vi "main_control_combo_backup.vi"(6 "read":bool=TRUE) -> (9 "chiller readout (temp)":string, 10 "bytes read":u32)   [LabVIEW 2019]
doc: "The Basic Serial Read and Write example performs a Serial Port Read, a Serial Port Write, or a combination of these actions. The user selects the actions (read or write) on the front panel. If both are selected, the VI will write the data first, read data, and then close the VISA session that is opened to the port. This VI will wait until the specified number of bytes is received at the port. Only the number of bytes specified will be read.\n\nINSTRUCTIONS:\n1) Select the serial resource and configuration parameters (baud rate, data bits, parity, stop bits, flow control).\n2) Select the operations to be performed. \n3) Connect the serial port to your device. If no device is available, perform a loopback test by doing one of the following. Short pins 2 and 3 on a RS-232 cable or short pin 4 to pin 8 and pin 5 to pin 9 on a RS-485/422 cable. \n4) Run the VI to see the data read. (The \"read string\" will match the \"string to write\" if a loopback test was performed.)\n\nNote: The parameters set for the serial port must match the parameters of the connected instrument or device. In this example, the bytes to read parameter specifies the number of bytes that the serial port reads. If there were more bytes at the port than the number specified in bytes to read, those bytes would not be read. Also, if you specify to read more bytes than the number of bytes actually read, you might receive a timeout error message.\n\nOn the block diagram, the Configure Serial Port VI sets the configuration parameters. The front panel displays the controls used to configure the basic parameters, such as baud rate, data bits, and parity. Constants configure the other parameters the user probably does not need set. After the VISA Configure Serial Port VI opens the VISA session and configures the port, the VI passes the VISA resource name to other VIs that perform operations on that VISA resource. The VISA Write function sends a command to the serial device and the VISA Read function returns data based on the command. The VISA Close function then closes the reference to the serial device. It is important to close the reference; otherwise communication through with that port through protocols other than VISA might not be possible."
uses:
  <vilib>/Instr/_visa.llb/VISA Configure Serial Port (Instr).vi
  Keithley/Keithley 24XX/Public/Data/Read (Single Point).vi
  <vilib>/Utility/file.llb/Read Delimited Spreadsheet (string).vi
  Keithley/Keithley 24XX/Keithley 24XX.lvlib
  <resource>/objmgr/ni.var.rc
panel:
  in  "read 4":bool
  in  "read \nrotronic log \nmanually":bool
  in  "times to run script":i32
  out "error out":errorcluster
  out "COMBO COMMAND":string
  out "manualDelta":bool
  out "delta readout":string
  in  "delay before read (ms) 4":u32=500
  in  "Combo Box 4":string(combo)
  in  "voltage delta":dbl
  out "delta command":string
  in  "write 4":bool
  in  "stop reading script":bool
  out "dewpoint":string
  out "temperature":string
  out "humidity":string
  out "n2 flow temperature":string
  out "dewpoint":string
  out "From Linux Box":string
  in  "Voltage Manual Range (1.0) 2":dbl=1.0
  in  "Current Manual Range (1.0) 2":dbl=1.0
  in  "Resistance Manual Range (1.0) 2":dbl=1.0
  in  "Enable Voltage Auto Range (T:Enable) 2":bool=TRUE
  in  "Enable Current Auto Range (T:Enable) 2":bool=TRUE
  in  "Enable Resistance Auto Range (T:Enable) 2":bool=TRUE
  out "Voltage 3":sgl
  out "Current 3":sgl
  out "Resistance 2":sgl
  out "Current Micro 2":sgl
  out "Command Log and Output":string
  out "all rows":string[][](array[string])
  out "current command":string[](array[string])
  in  "file path (dialog if empty) 2":path
  in  "Read Script":bool
  out "relay TTi":errorcluster
  out "bytes read 3":u32
  out "inverter readout":string
  in  "read 3":bool=TRUE
  in  "delay before read (ms) 3":u32=500
  in  "Combo Box 3":string(combo)="VO?\n"
  in  "voltage or current 2":dbl
  out "string from combo 3":string
  in  "write 3":bool
  out "LV TTi":errorcluster
  out "bytes read 2":u32
  out "LVPS reaout":string
  in  "read 2":bool=TRUE
  in  "delay before read (ms) 2":u32=500
  in  "Combo Box 2":string(combo)="VO?\n"
  in  "voltage or current":dbl
  in  "write 2":bool
  in  "write":bool
  out "string from combo":string
  in  "Temperature":dbl
  in  "Combo Box":string(combo)
  out "Chiller":errorcluster
  out "N2 temperature > dew point + 5C":bool
  in  "File Path of rotonic datalog":path
  out "time humidity temporature dewpoint":string[](array[string])
  in  "Quit":bool
  in  "delay before read (ms)":u32=500
  # "Kiethley Powersupply"
  # "µA"
  # "Delta powersupply Interface"
  # "TTi LV powersupply Interface for the relay polarity control\nCOM 4 is default"
  # "Medical Chiller Interface\nCOM 6 is default"
  # "TTi LV powersupply Interface\nCOM 5 is default"
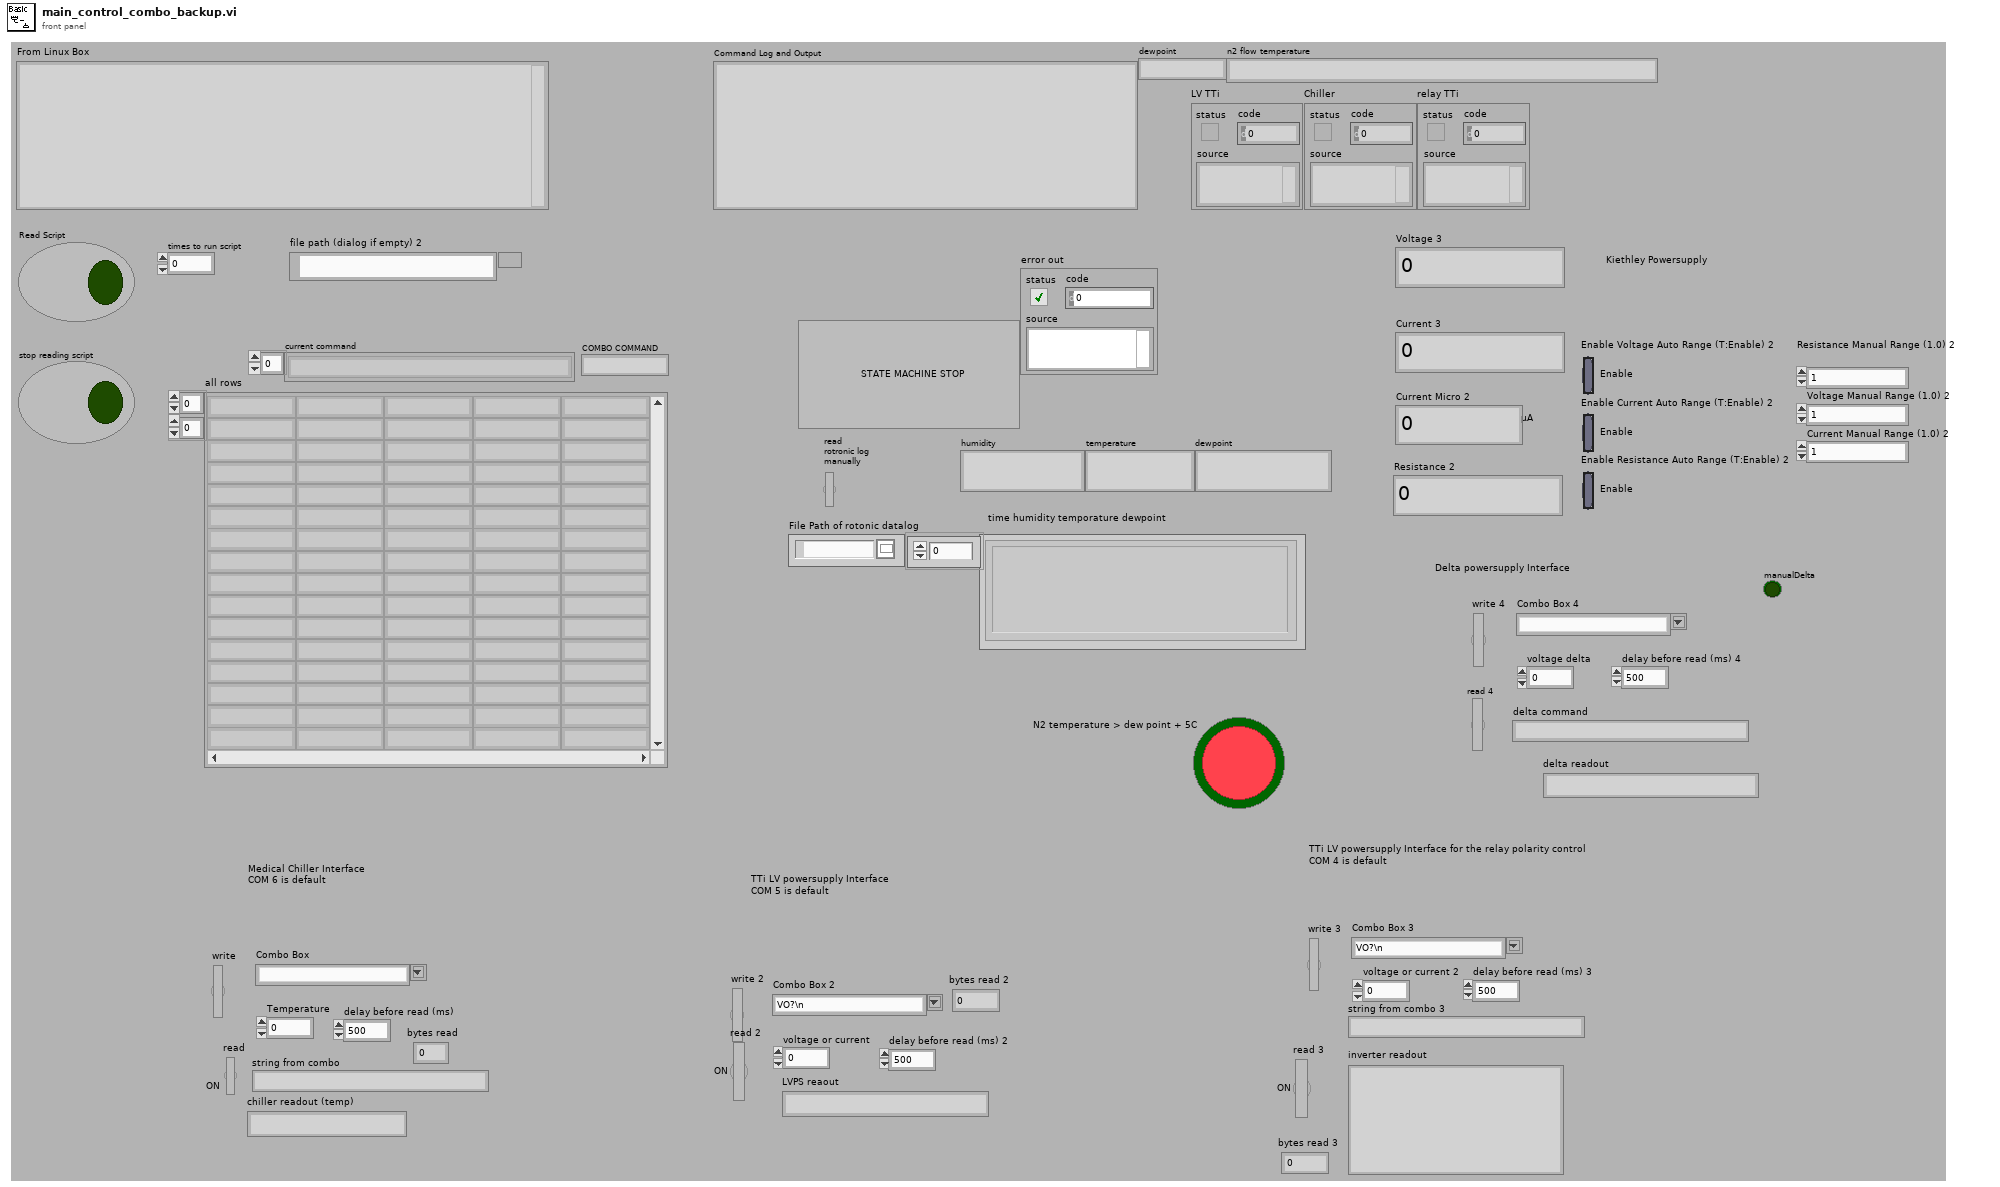
[diagram p1: front panel]
types:
  T1 = cluster{"Baud Rate":u32, "Parity":u16, "Data Bits":u16, "Stop Bits":u16, "Flow Control":u16}
  T2 = enum16{"open", "replace", "create", "open or create", "replace or create", "replace or create with confirmation"}
  T3 = typedef "Semaphore RefNum" = refnum<k1>
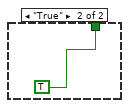
[diagram p2: hidden frame]
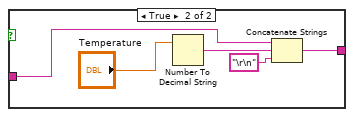
[diagram p5: hidden frame]
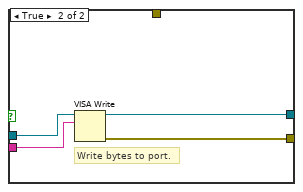
[diagram p6: hidden frame]
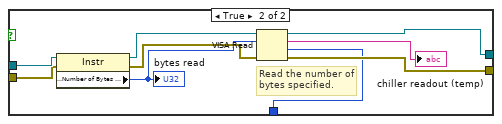
[diagram p7: hidden frame]
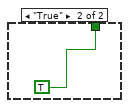
[diagram p8: hidden frame]
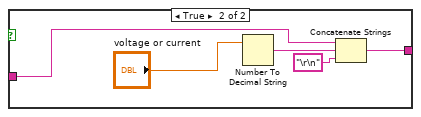
[diagram p10: hidden frame]
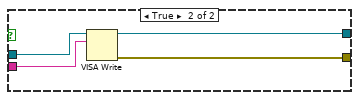
[diagram p11: hidden frame]
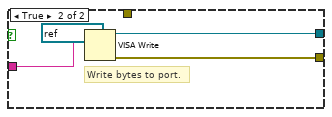
[diagram p16: hidden frame]
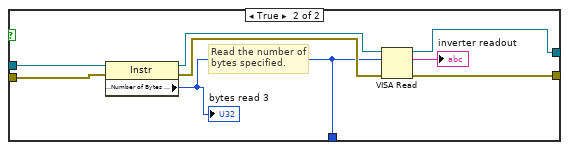
[diagram p17: hidden frame]
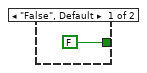
[diagram p18: hidden frame]
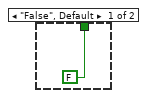
[diagram p19: hidden frame]
diagram:
  # "First save permanent values in non-volatile memory via NI - Max and the *SAV after setting it via SO:VO:MA 52 and SO:CU:MA 30    !"
  n1 = flat-sequence {
    tunnel: [w20] -> w13
    tunnel: [w34] -> w12
    tunnel: [w22] -> w11
    tunnel: [w28] -> w10
    tunnel: [w27] -> w9
    tunnel: [w23] -> w8
    tunnel: [w23] -> w7
    tunnel: [w19] -> w6
    tunnel: [w18] -> w5
    tunnel: [w17] -> w4
    tunnel: [w19] -> w3
    tunnel: [w18] -> w2
    tunnel: [w17] -> w1
    tunnel: [w54] -> w16
    tunnel: [w53] -> w14
    tunnel: w13 -> [w52]
    tunnel: w12 -> [_]
    tunnel: w11 -> [w51]
    tunnel: w10 -> [w49]
    tunnel: w9 -> [w50]
    tunnel: w8 -> [w48]
    tunnel: w7 -> [w47]
    tunnel: w6 -> [w46]
    tunnel: w5 -> [w45]
    tunnel: w4 -> [w44]
    tunnel: w3 -> [w43]
    tunnel: w2 -> [w42]
    tunnel: w1 -> [w41]
    tunnel: w16 -> [w668]
    tunnel: w14 -> [w667]
    frame #0 {
      w21 = refnum<visa-resource-name> "COM4" ("VISA resource name")
      w26 = u32 3000  # timeout (10sec)
      w25 = FALSE  # Enable Termination Char (T)
      w29 = u32 3000  # timeout (10sec)
      w31 = FALSE  # Enable Termination Char (T)
      w32 = u32 3000  # timeout (10sec)
      w35 = FALSE  # Enable Termination Char (T)
      w36 = u32 3000  # timeout (10sec)
      n2 = call "Initialize.vi"("Serial Configuration"=T1 {"Baud Rate"=9600, "Parity"=0, "Data Bits"=8, "Stop Bits"=10, "Flow Control"=1}, "Reset (True)"=FALSE, "VISA resource name"=refnum<visa-resource-name> "COM1" ("VISA resource name 4")) -> ()  [unwired: 7 in, 2 out]
      n3 = local write "COMBO COMMAND"("" ("COMBO COMMAND")) -> ()
      n4 = VISA Open(timeout (0)=w29, VISA resource name=refnum<visa-resource-name> "GPIB0::8::INSTR") -> (VISA resource name=w28:refnum<visa-resource-name>, error out=w27:errorcluster)  [unwired: 3 in]
      n5 = call-poly "VISA Configure Serial Port"("VISA resource name"=refnum<visa-resource-name> "COM5", "timeout (10sec)"=w32, "Enable Termination\nChar (T)"=w31) -> ("VISA resource name out"=w22:refnum<visa-resource-name>)  [unwired: 11 in, 1 out]
      n6 = call <vilib>:"Obtain Semaphore Reference.vi"("name (unnamed)"=w21) -> ("semaphore"=w18:T3)  [unwired: 4 in, 2 out]
      n7 = call-poly "VISA Configure Serial Port"("VISA resource name"=w21, "timeout (10sec)"=w26, "Enable Termination\nChar (T)"=w25) -> ()  [unwired: 11 in, 2 out]
      n8 = call-poly "VISA Configure Serial Port"("VISA resource name"=refnum<visa-resource-name> "COM6", "timeout (10sec)"=w36, "Enable Termination\nChar (T)"=w35) -> ("VISA resource name out"=w20:refnum<visa-resource-name>, "error out"=w34:errorcluster)  [unwired: 11 in]
      n9 = call <vilib>:"Obtain Semaphore Reference.vi"("name (unnamed)"=w22) -> ("semaphore"=w17:T3)  [unwired: 4 in, 2 out]
      n10 = call <vilib>:"Obtain Semaphore Reference.vi"("name (unnamed)"=w20) -> ("semaphore"=w19:T3)  [unwired: 4 in, 2 out]
      n11 = call <vilib>:"Obtain Semaphore Reference.vi"("name (unnamed)"=w28) -> ("semaphore"=w23:T3)  [unwired: 4 in, 2 out]
    }
    frame #1 {
      # "Disable Output"
      # "State machine for iterating through commands from table"
      n12 = while {
        tunnel: w48 -> [w367]
        tunnel: w46 -> [w366]
        tunnel: w45 -> [w365]
        tunnel: w44 -> [w364]
        stop <- w369 stop-if-true
        # "LV TTi SEH"
        # "inverter"
        # "chiller"
        # "DeltaRef"
        n13 = local read "Quit"() -> (w369:bool)
        n14 = case shown="True" "Read Script" {
          tunnel: "times to run script" -> [_ w375]
          tunnel: w367 -> [_ w374]
          tunnel: w366 -> [_ w373]
          tunnel: w365 -> [_ w372]
          tunnel: w364 -> [_ w371]
          frame False {
          }
          frame True {
            n15 = Get Date/Time String() -> (date string=w398:string, time string=w396:string)  [unwired: 3 in]
            n16 = Search and Replace String(replace all?=TRUE ("replace all? (F)"), input string=w398, search string="/", replace string="_" ("replace string (\"\")")) -> (result string=w397:string)  [unwired: 4 in, 3 out]
            n17 = Search and Replace String(input string=w396, search string=":", replace string="" ("replace string (\"\")")) -> (result string=w395:string)  [unwired: 5 in, 3 out]
            n18 = Concatenate Strings("C:\\Users\\CMSOTDSF.CERN\\ExecutedCommands\\" ("string"), "command_log_" ("string"), w397, "_" ("string"), w395, ".txt" ("string")) -> (w394:string)
            n19 = String To Path(string=w394) -> (path=w384:path)
            n20 = Open/Create/Replace File(file path (use dialog)=w384, operation (0:open)=T2."replace or create") -> (refnum out=w383:refnum<file>)  [unwired: 4 in, 2 out]
            n21 = Concatenate Strings("Command Log Header for Executed CSV commands " ("text"), "\r\n") -> (w376:string)
            n22 = Set File Position(offset (in bytes) (0)=i64 0, refnum=w383, from (0:start)=enum16{"start", "end", "current"}."end") -> (refnum out=w380:refnum<file>)  [unwired: 1 in, 1 out]
            n23 = Write to Text File(file (use dialog)=w380, text=w376) -> ()  [unwired: 2 in, 3 out]
            n24 = flat-sequence {
              tunnel: w384 -> [w404]
              tunnel: w375 -> [w403]
              tunnel: w374 -> [w402]
              tunnel: w373 -> [w401]
              tunnel: w372 -> [w400]
              tunnel: w371 -> [w399]
              frame #0 {
                n25 = for {
                  N: w403 -> [_]
                  tunnel: w404 -> [w409]
                  tunnel: w402 -> [w408]
                  tunnel: w401 -> [w407]
                  tunnel: w400 -> [w406]
                  tunnel: w399 -> [w405]
                  n26 = flat-sequence {
                    tunnel: ["file path (dialog if empty) 2"] -> w412
                    tunnel: [w415] -> w411
                    tunnel: [w413] -> w410
                    tunnel: w409 -> [w413]
                    tunnel: w412 -> [_]
                    tunnel: w411 -> [w422]
                    tunnel: w410 -> [w421]
                    tunnel: w408 -> [w420]
                    tunnel: w407 -> [w419]
                    tunnel: w406 -> [w418]
                    tunnel: w405 -> [w417]
                    frame #0 {
                      # "read table from CSV"
                      n27 = call-poly <vilib>:"Read Delimited Spreadsheet.vi"("file path (dialog if empty)"="file path (dialog if empty) 2", "delimiter (\\t)"="," ("delimiter (\\t)")) -> ("all rows"=w415:string[][])  [unwired: 8 in, 5 out]
                    }
                    frame #1 {
                      n28 = Array Size(array=w422) -> (size(s)=w425:i32[])
                      n29 = Index Array(array=w425, index #1=0 ("index"), index #2=1 ("index")) -> (element #1=w426:i32)  [unwired: 1 out]
                      n30 = for {
                        N: w426 -> [_]
                        tunnel: w422 -> [w454] mode=indexing
                        tunnel: w421 -> [w442]
                        tunnel: w420 -> [w430]
                        tunnel: w419 -> [w429]
                        tunnel: w418 -> [w428]
                        tunnel: w417 -> [w427]
                        i -> [w439]
                        stop <- w448 stop-if-true
                        n31 = local read "Quit"() -> (w450:bool)
                        n32 = Array Subset(array=w454) -> (w451:string[])  [unwired: 2 in]
                        "current command" <- w451
                        n33 = Or(x=w450, y="stop reading script") -> (x .or. y?=w448:bool)
                        n34 = Array Size(array=w451) -> (size(s)=w453:i32)
                        n35 = Index Array(array=w451, index=0) -> (element=w431:string)
                        "COMBO COMMAND" <- w431
                        n36 = for {
                          N: w453 -> [_]
                          tunnel: w451 -> [w614]
                          tunnel: [w615] -> w432 mode=indexing
                          i -> [w617]
                          n37 = Add(x=w617, y=1) -> (x+y=w613:i32)
                          n38 = Index Array(array=w614, index=w613) -> (element=w612:string)
                          n39 = Wait Until Next ms Multiple(millisecond multiple=u32 1000) -> ()  [unwired: 1 out]
                          n40 = Concatenate Strings(w612, "   " ("string")) -> (w615:string)
                        }
                        n41 = case shown="\"setDeltaPS\"" w431 {
                          tunnel: w451 -> [w462 w474 w495 w513 w548 w576 _ _]
                          tunnel: [w455 w471 w493 w505 w541 w572 _ w585] -> w440
                          tunnel: w430 -> [_ _ w487 w504 _ _ _ _]
                          tunnel: w429 -> [_ _ _ _ w540 _ _ _]
                          tunnel: w428 -> [_ _ _ w500 _ _ _ _]
                          tunnel: w427 -> [_ w463 _ _ _ _ _ _]
                          frame "wait", Default {
                            n42 = Array Subset(array=w462, index=1) -> (w460:string[])  [unwired: 1 in]
                            n43 = Index Array(array=w460, index=0) -> (element=w456:string)
                            n44 = Decimal String To Number(string=w456) -> (number=w458:i32)  [unwired: 2 in, 1 out]
                            n45 = Wait (ms)(milliseconds to wait=w458) -> ()  [unwired: 1 out]
                            n46 = Concatenate Strings("Wait for ", w456) -> (w455:string)
                          }
                          frame "setLVPS" {
                            # "Write bytes to port."
                            # "MUST specify codes display with single \"\\\""
                            # "Configure Serial port (baud rate,\ndata bits, parity, stop bits and flow control)."
                            n47 = Array Subset(array=w474, index=1) -> (w479:string[])  [unwired: 1 in]
                            n48 = Index Array(array=w479, index #1=0 ("index"), index #2=1 ("index")) -> (element #1=w476:string)  [unwired: 1 out]
                            n49 = Decimal String To Number(string=w476) -> (number=w473:i32)  [unwired: 2 in, 1 out]
                            n50 = To Double Precision Float(number=w473) -> (double precision float=w470:dbl)
                            n51 = case shown="0, Default" w470 {
                              tunnel: ["OP 0\n" ("Combo Box 4") "OP 1\n" ("Combo Box 4")] -> w469
                              tunnel: ["0" ("Combo Box 4") "11" ("Combo Box 4")] -> w467
                              frame 0, Default {
                              }
                              frame 1 {
                              }
                            }
                            n52 = call <vilib>:"Acquire Semaphore.vi"("semaphore"=w463) -> ("error out"=w465:errorcluster, "semaphore out"=w466:T3)  [unwired: 4 in, 1 out]
                            n53 = VISA Write(VISA resource name=refnum<visa-resource-name> "COM5", write buffer=w469, error in (no error)=w465) -> (error out=w464:errorcluster)  [unwired: 2 out]
                            n54 = call <vilib>:"Release Semaphore.vi"("error in (no error)"=w464, "semaphore"=w466) -> ()  [unwired: 4 in, 2 out]
                            n55 = Concatenate Strings("we just set the LV PS voltage to ", w467) -> (w471:string)
                          }
                          frame "setDeltaPS" {
                            # "MUST specify codes display with single \"\\\""
                            # "Configure Serial port (baud rate,\ndata bits, parity, stop bits and flow control)."
                            n56 = Array Subset(array=w495, index=1) -> (w499:string[])  [unwired: 1 in]
                            n57 = Index Array(array=w499, index #1=0 ("index"), index #2=1 ("index")) -> (element #1=w488:string)  [unwired: 1 out]
                            n58 = call <vilib>:"Acquire Semaphore.vi"("semaphore"=w487) -> ("error out"=w486:errorcluster, "semaphore out"=w484:T3)  [unwired: 4 in, 1 out]
                            n59 = Concatenate Strings("SOUR:VO " ("format string"), w488, "\n" ("string")) -> (w490:string)
                            n60 = VISA Write(VISA resource name=refnum<visa-resource-name> "GPIB0::8::INSTR", write buffer=w490, error in (no error)=w486) -> (error out=w485:errorcluster)  [unwired: 2 out]
                            n61 = call <vilib>:"Release Semaphore.vi"("error in (no error)"=w485, "semaphore"=w484) -> ()  [unwired: 4 in, 2 out]
                            n62 = Concatenate Strings("we just set the Delta voltage to ", w488) -> (w493:string)
                          }
                          frame "setInverter" {
                            # "MUST specify codes display with single \"\\\""
                            # "Configure Serial port (baud rate,\ndata bits, parity, stop bits and flow control)."
                            n63 = Array Subset(array=w513, index=1) -> (w518:string[])  [unwired: 1 in]
                            n64 = Index Array(array=w518, index #1=0 ("index"), index #2=1 ("index")) -> (element #1=w515:string)  [unwired: 1 out]
                            n65 = Decimal String To Number(string=w515) -> (number=w512:i32)  [unwired: 2 in, 1 out]
                            n66 = To Double Precision Float(number=w512) -> (double precision float=w506:dbl)
                            n67 = call <vilib>:"Acquire Semaphore.vi"("semaphore"=w504) -> ("error out"=w503:errorcluster, "semaphore out"=w501:T3)  [unwired: 4 in, 1 out]
                            n68 = call "deltaPS.vi"("error in (no error)"=w503, "VISA Refnum in"=refnum<visa-resource-name> "GPIB0::8::INSTR" ("VISA resource name")) -> ("error out"=w502:errorcluster, "DeltaPS"=w507:string)  [unwired: 8 in]
                            n69 = Decimal String To Number(string=w507) -> (number=w508:i32)  [unwired: 2 in, 1 out]
                            n70 = Less?(x=w508, y=3.0) -> (x < y?=w510:bool)
                            n71 = case shown="False" w510 {
                              tunnel: w506 -> [_ w530]
                              tunnel: w507 -> [w521 _]
                              tunnel: [w520 w527] -> w505
                              tunnel: w500 -> [_ w523]
                              frame False {
                                n72 = local write "stop reading script"(TRUE ("stop reading script")) -> ()
                                n73 = Concatenate Strings("Dangerous polarity switching   Delta PS too high:    ", w521) -> (w520:string)
                                n74 = call "Send Email"("Message"=w520) -> ()  [unwired: 10 in, 1 out]
                              }
                              frame True {
                                # "Write bytes to port."
                                n75 = case shown="1" w530 {
                                tunnel: ["OP 0\n" ("Combo Box 4") "OP 1\n" ("Combo Box 4")] -> w532
                                tunnel: ["0" ("Combo Box 4") "10" ("Combo Box 4")] -> w528
                                frame 0, Default {
                                }
                                frame 1 {
                                }
                                }
                                n76 = call <vilib>:"Acquire Semaphore.vi"("semaphore"=w523) -> ("error out"=w526:errorcluster, "semaphore out"=w524:T3)  [unwired: 4 in, 1 out]
                                n77 = VISA Write(VISA resource name=refnum<visa-resource-name> "COM4", write buffer=w532, error in (no error)=w526) -> (error out=w525:errorcluster)  [unwired: 2 out]
                                n78 = Concatenate Strings("we just set the Inverter voltage to ", w528) -> (w527:string)
                                n79 = call <vilib>:"Release Semaphore.vi"("error in (no error)"=w525, "semaphore"=w524) -> ()  [unwired: 4 in, 2 out]
                              }
                            }
                            n80 = call <vilib>:"Release Semaphore.vi"("error in (no error)"=w502, "semaphore"=w501) -> ()  [unwired: 4 in, 2 out]
                          }
                          frame "setChiller" {
                            # "Write bytes to port."
                            # "MUST specify codes display with single \"\\\""
                            # "Configure Serial port (baud rate,\ndata bits, parity, stop bits and flow control)."
                            n81 = Array Subset(array=w548, index=1) -> (w552:string[])  [unwired: 1 in]
                            n82 = Index Array(array=w552, index #1=0 ("index"), index #2=1 ("index")) -> (element #1=w543:string, element #2=w545:string)
                            n83 = Decimal String To Number(string=w545) -> (number=w544:i32)  [unwired: 2 in, 1 out]
                            n84 = To Double Precision Float(number=w544) -> (double precision float=w542:dbl)
                            n85 = call <vilib>:"Acquire Semaphore.vi"("semaphore"=w540) -> ("error out"=w539:errorcluster, "semaphore out"=w538:T3)  [unwired: 4 in, 1 out]
                            n86 = case shown="\"stop\", Default" w543 {
                              tunnel: ["STOP\n" ("Combo Box 4") "START\n" ("Combo Box 4") w561] -> w547
                              tunnel: w542 -> [_ _ w560]
                              tunnel: ["we just stop the chiller" "we just start the chiller" w557] -> w541
                              frame "stop", Default {
                              }
                              frame "start" {
                              }
                              frame "settemp" {
                                n87 = Number To Decimal String(number=w560) -> (decimal integer string=w559:string)  [unwired: 1 in]
                                n88 = Concatenate Strings("OUT_SP_00_" ("Combo Box 4"), w559, "\r\n" ("string")) -> (w561:string)
                                n89 = Concatenate Strings("we just set the Chiller temperature to ", w559) -> (w557:string)
                              }
                            }
                            n90 = VISA Write(VISA resource name=refnum<visa-resource-name> "COM6", write buffer=w547, error in (no error)=w539) -> (error out=w537:errorcluster)  [unwired: 2 out]
                            n91 = call <vilib>:"Release Semaphore.vi"("error in (no error)"=w537, "semaphore"=w538) -> ()  [unwired: 4 in, 2 out]
                          }
                          frame "keithleynew" {
                            w564 = u16 0 items=["Voltage", "Current"] ("Source Mode  (0: Voltage)")
                            # "Configure each of the three measurements. settings"
                            n92 = Array Subset(array=w576, index=1) -> (w579:string[])  [unwired: 1 in]
                            n93 = Index Array(array=w579, index #1=0 ("index"), index #2=1 ("index")) -> (element #1=w573:string)  [unwired: 1 out]
                            n94 = Decimal String To Number(string=w573) -> (number=w575:i32)  [unwired: 2 in, 1 out]
                            n95 = To Double Precision Float(number=w575) -> (double precision float=w570:dbl)
                            n96 = Concatenate Strings("we just set the keithley voltage to ", w573) -> (w572:string)
                            n97 = call "Configure Output.vi"("Source Mode  (0: Voltage)"=w564, "Compliance  Level (0.1)"=1e-05, "Output Level (0)"=w570, "VISA resource name"=refnum<visa-resource-name> "COM1") -> ("error out"=w568:errorcluster, "VISA resource name out"=w569:refnum<visa-resource-name>)  [unwired: 6 in]
                            n98 = call "Enable Output.vi"("error in (no error)"=w568, "Enable Output (T: Enable)"=TRUE, "VISA resource name"=w569) -> ()  [unwired: 7 in, 2 out]
                          }
                          frame "closekeithley" {
                            n99 = call "Enable Output.vi"("Enable Output (T: Enable)"=FALSE, "VISA resource name"=refnum<visa-resource-name> "COM1") -> ("error out"=w581:errorcluster, "VISA resource name out"=w582:refnum<visa-resource-name>)  [unwired: 8 in]
                            n100 = call "Close.vi"("error in (no error)"=w581, "VISA resource name"=w582) -> ("error out"=w584:errorcluster)  [unwired: 9 in]
                            n101 = call <vilib>:"Simple Error Handler.vi"("error in (no error)"=w584) -> ()  [unwired: 4 in, 5 out]
                          }
                          frame "2sCalibration" {
                            # "C:\\Users\\CMSOTDSF.CERN\\2sCalibrationOut"
                            # "run a windows batch file that will call ssh command with an INPUT bash script\nThe input bash script will run the 2s calibration and is located here:\nC:\\Users\\CMSOTDSF.CERN\\cc7.sh"
                            n102 = flat-sequence {
                              tunnel: [w588] -> w586
                              tunnel: w586 -> [w594]
                              tunnel: [w593] -> w585
                              frame #0 {
                                n103 = call <vilib>:"System Exec.vi"("run minimized? (F)"=TRUE, "working directory"=path "C:/Users/CMSOTDSF.CERN/OpenSSH", "command line"="cmd /c C:\\Users\\CMSOTDSF.CERN\\windows_cc7.bat") -> ("standard error"=w589:string, "standard output"=w590:string)  [unwired: 5 in, 2 out]
                                "From Linux Box" <- w590
                                n104 = Concatenate Strings(w590, w589) -> (w588:string)
                              }
                              frame #1 {
                                n105 = Get Date/Time String() -> (date string=w605:string, time string=w607:string)  [unwired: 3 in]
                                n106 = Search and Replace String(input string=w607, search string=":", replace string="" ("replace string (\"\")")) -> (result string=w608:string)  [unwired: 5 in, 3 out]
                                n107 = Search and Replace String(replace all?=TRUE ("replace all? (F)"), input string=w605, search string="/", replace string="_" ("replace string (\"\")")) -> (result string=w606:string)  [unwired: 4 in, 3 out]
                                n108 = Concatenate Strings("C:\\Users\\CMSOTDSF.CERN\\2sCalibrationOut\\" ("string"), "2scalibration_" ("string"), w606, "_" ("string"), w608, ".txt" ("string")) -> (w609:string)
                                n109 = String To Path(string=w609) -> (path=w610:path)
                                n110 = Concatenate Strings("2S Calibration done output is saved to: ", w609) -> (w593:string)
                                n111 = Write to Text File(file (use dialog)=w610, text=w594) -> ()  [unwired: 2 in, 3 out]
                              }
                            }
                          }
                        }
                        "Command Log and Output" <- w440
                        n112 = Add(x=w439, y=1) -> (x+y=w437:i32)
                        n113 = Number To Decimal String(number=w437) -> (decimal integer string=w436:string)  [unwired: 1 in]
                        n114 = Open/Create/Replace File(file path (use dialog)=w442, operation (0:open)=T2."open") -> (refnum out=w443:refnum<file>)  [unwired: 4 in, 2 out]
                        n115 = Concatenate Strings(w436, "  " ("string"), w431, "  " ("string"), w432, "\r\n") -> (w441:string)
                        n116 = Set File Position(offset (in bytes) (0)=i64 0, refnum=w443, from (0:start)=enum16{"start", "end", "current"}."end") -> (refnum out=w445:refnum<file>)  [unwired: 1 in, 1 out]
                        n117 = Write to Text File(file (use dialog)=w445, text=w441) -> ()  [unwired: 2 in, 3 out]
                      }
                      "all rows" <- w422
                    }
                  }
                }
              }
              frame #1 {
                n118 = local write "COMBO COMMAND"("" ("COMBO COMMAND")) -> ()
                n119 = invoke on="Read Script" class="Bool (strict)" method="Reinit To Default"() -> ()  [unwired: 3 in, 3 out]
                n120 = invoke on="stop reading script" class="Bool (strict)" method="Reinit To Default"() -> ()  [unwired: 3 in, 3 out]
              }
            }
          }
        }
      }
      n121 = while {
        tunnel: w49 -> [_]
        tunnel: w50 -> [_]
        tunnel: w47 -> [w253]
        stop <- w267 stop-if-true
        w256 = "True" ("replace string (\"\")")
        n122 = local read "COMBO COMMAND"() -> (w260:string)
        n123 = Search and Replace String(input string=w260, search string="setInverter", replace string=w256) -> (result string=w265:string)  [unwired: 5 in, 3 out]
        n124 = Search and Replace String(input string=w260, search string="setDeltaPS", replace string=w256) -> (result string=w262:string)  [unwired: 5 in, 3 out]
        n125 = case shown="\"True\"" w265 {
          tunnel: [FALSE TRUE] -> w266
          frame "False", Default {
          }
          frame "True" {
          }
        }
        n126 = case shown="\"False\", Default" w262 {
          tunnel: [FALSE TRUE] -> w263
          frame "False", Default {
          }
          frame "True" {
          }
        }
        n127 = local read "Quit"() -> (w264:bool)
        n128 = call <vilib>:"Acquire Semaphore.vi"("semaphore"=w253) -> ("error out"=w254:errorcluster, "semaphore out"=w251:T3)  [unwired: 4 in, 1 out]
        n129 = Or(x=w263, y=w264) -> (x .or. y?=w259:bool)
        n130 = Or(x=w259, y=w266) -> (x .or. y?=w258:bool)
        n131 = Not(x=w258) -> (.not. x?=w261:bool)
        "manualDelta" <- w261
        n132 = case shown="True" w261 {
          tunnel: w254 -> [w270 w276]
          tunnel: [w270 w275] -> w252
          frame False {
          }
          frame True {
            # "delta"
            # "Configure Serial port (baud rate,\ndata bits, parity, stop bits and flow control)."
            n133 = Match True/False String(2:"" ("false string"), 3:"SOUR:VO " ("format string"), 4:"Combo Box 4") -> (0:w281:bool)  [unwired: 1 out]
            n134 = case shown="True" w281 {
              tunnel: [w289 w292] -> w278
              tunnel: "Combo Box 4" -> [w289 w291]
              frame False {
              }
              frame True {
                n135 = Number To Decimal String(number="voltage delta") -> (decimal integer string=w294:string)  [unwired: 1 in]
                n136 = Concatenate Strings(w291, w294, "\n" ("string")) -> (w292:string)
              }
            }
            "delta command" <- w278
            n137 = case shown="True" "write 4" {
              tunnel: [w300 w306] -> w286
              tunnel: [w301 w305] -> w284
              tunnel: w278 -> [_ w304]
              tunnel: w276 -> [w298 _]
              frame False {
                n138 = VISA Write(VISA resource name=refnum<visa-resource-name> "GPIB0::8::INSTR", write buffer="ME:VO?\n", error in (no error)=w298) -> (VISA resource name out=w301:refnum<visa-resource-name>, error out=w300:errorcluster)  [unwired: 1 out]
              }
              frame True {
                # "Write bytes to port."
                n139 = VISA Write(VISA resource name=refnum<visa-resource-name> "GPIB0::8::INSTR", write buffer=w304) -> (VISA resource name out=w305:refnum<visa-resource-name>, error out=w306:errorcluster)  [unwired: 1 in, 1 out]
              }
            }
            n140 = stacked-sequence {
              tunnel: w286 -> [w297]
              tunnel: [w297] -> w285
              tunnel: w284 -> [w296]
              tunnel: [w296] -> w283
              frame #0 {
                n141 = Wait (ms)(milliseconds to wait="delay before read (ms) 4") -> ()  [unwired: 1 out]
              }
            }
            n142 = case shown="True" "read 4" {
              tunnel: w285 -> [w309 w311]
              tunnel: [w309 w316] -> w275
              tunnel: [w308 w315] -> _
              tunnel: w283 -> [w308 w313]
              tunnel: [u32 10 ("return count") w310] -> w273
              frame False {
              }
              frame True {
                # "Read the number of bytes specified."
                n143 = VISA Read(VISA resource name=w313, byte count=u32 1024, error in (no error)=w311) -> (VISA resource name out=w315:refnum<visa-resource-name>, read buffer=→"delta readout":string, return count=w310:u32, error out=w316:errorcluster)
              }
            }
            n144 = Equal?(x=w273, y=0.0) -> (x = y?=w272:bool)
            n145 = case shown="True" w272 {
              frame False {
              }
              frame True {
                n146 = call "delta email"() -> ()  [unwired: 11 in, 1 out]
                n147 = local write "stop reading script"(TRUE ("stop reading script")) -> ()
                n148 = local write "write 4"(TRUE ("write 4")) -> ()
              }
            }
          }
        }
        n149 = local read "Quit"() -> (w267:bool)
        n150 = call <vilib>:"Release Semaphore.vi"("error in (no error)"=w252, "semaphore"=w251) -> ()  [unwired: 4 in, 2 out]
      }
      n151 = while {
        stop <- "Quit" stop-if-true
      }
      n152 = while {
        tunnel: w51 -> [w139]
        tunnel: [w140] -> w54
        tunnel: w41 -> [w128]
        stop <- w138 stop-if-true
        n153 = local read "COMBO COMMAND"() -> (w130:string)
        n154 = call <vilib>:"Acquire Semaphore.vi"("semaphore"=w128) -> ("error out"=w127:errorcluster, "semaphore out"=w125:T3)  [unwired: 4 in, 1 out]
        n155 = Search and Replace String(input string=w130, search string="setLVPS", replace string="True" ("replace string (\"\")")) -> (result string=w135:string)  [unwired: 5 in, 3 out]
        n156 = case shown="\"False\", Default" w135 {
          tunnel: [FALSE TRUE] -> w136
          frame "False", Default {
          }
          frame "True" {
          }
        }
        n157 = local read "Quit"() -> (w137:bool)
        n158 = Or(x=w136, y=w137) -> (x .or. y?=w132:bool)
        n159 = Not(x=w132) -> (.not. x?=w131:bool)
        n160 = case shown="True" w131 {
          tunnel: [w143 w159] -> w126
          tunnel: [w144 w158] -> w140
          tunnel: w139 -> [w144 w157]
          tunnel: w127 -> [w143 w145]
          frame False {
          }
          frame True {
            # "TTi SEH PS LV"
            n161 = Match True/False String(2:"" ("false string"), 3:"OUT_SP_00_" ("format string"), 4:"Combo Box 2") -> (0:w150:bool)  [unwired: 1 out]
            n162 = case shown="False" w150 {
              tunnel: [w160 w163] -> w147
              tunnel: "Combo Box 2" -> [w160 w162]
              frame False {
              }
              frame True {
                n163 = Number To Decimal String(number="voltage or current") -> (decimal integer string=w165:string)  [unwired: 1 in]
                n164 = Concatenate Strings(w162, w165, "\r\n" ("string")) -> (w163:string)
              }
            }
            n165 = case shown="False" "write 2" {
              tunnel: [w170 w177] -> w155
              tunnel: w157 -> [w172 w176]
              tunnel: [w171 w175] -> w153
              tunnel: w147 -> [_ w174]
              tunnel: w145 -> [w169 _]
              frame False {
                n166 = VISA Write(VISA resource name=w172, write buffer="VO?\n", error in (no error)=w169) -> (VISA resource name out=w171:refnum<visa-resource-name>, error out=w170:errorcluster)  [unwired: 1 out]
              }
              frame True {
                n167 = VISA Write(VISA resource name=w176, write buffer=w174) -> (VISA resource name out=w175:refnum<visa-resource-name>, error out=w177:errorcluster)  [unwired: 1 in, 1 out]
              }
            }
            n168 = stacked-sequence {
              tunnel: w155 -> [w168]
              tunnel: [w168] -> w154
              tunnel: w153 -> [w167]
              tunnel: [w167] -> w152
              frame #0 {
                n169 = Wait (ms)(milliseconds to wait="delay before read (ms) 2") -> ()  [unwired: 1 out]
              }
            }
            n170 = case shown="True" "read 2" {
              tunnel: w154 -> [w179 w183]
              tunnel: [w179 w187] -> w159
              tunnel: [w178 w186] -> w158
              tunnel: w152 -> [w178 w185]
              frame False {
              }
              frame True {
                # "Read the number of bytes specified."
                n171 = property class="Instr"(reference=w185, error in=w183) -> (reference out=w184:refnum<visa-resource-name>, error out=w182:errorcluster, "Serial Settings:Number of Bytes at Serial Port"=w181:u32)
                "bytes read 2" <- w181
                n172 = VISA Read(VISA resource name=w184, byte count=w181, error in (no error)=w182) -> (VISA resource name out=w186:refnum<visa-resource-name>, read buffer=→"LVPS reaout":string, error out=w187:errorcluster)  [unwired: 1 out]
              }
            }
          }
        }
        n173 = call <vilib>:"Release Semaphore.vi"("error in (no error)"=w126, "semaphore"=w125) -> ()  [unwired: 4 in, 2 out]
        n174 = local read "Quit"() -> (w138:bool)
        n175 = Wait Until Next ms Multiple(millisecond multiple=u32 1000) -> ()  [unwired: 1 out]
      }
      n176 = while {
        tunnel: w42 -> [w191]
        stop <- w200 stop-if-true
        # "TTi Inverter for Relay"
        n177 = local read "COMBO COMMAND"() -> (w198:string)
        n178 = call <vilib>:"Acquire Semaphore.vi"("semaphore"=w191) -> ("error out"=w188:errorcluster, "semaphore out"=w190:T3)  [unwired: 4 in, 1 out]
        n179 = Search and Replace String(input string=w198, search string="setInverter", replace string="True" ("replace string (\"\")")) -> (result string=w194:string)  [unwired: 5 in, 3 out]
        n180 = case shown="\"True\"" w194 {
          tunnel: [FALSE TRUE] -> w195
          frame "False", Default {
          }
          frame "True" {
          }
        }
        n181 = local read "Quit"() -> (w196:bool)
        n182 = Or(x=w195, y=w196) -> (x .or. y?=w197:bool)
        n183 = Not(x=w197) -> (.not. x?=w199:bool)
        n184 = case shown="True" w199 {
          tunnel: [w201 w206] -> w189
          tunnel: w188 -> [w201 w205]
          frame False {
          }
          frame True {
            # "Configure Serial port (baud rate,\ndata bits, parity, stop bits and flow control)."
            n185 = Match True/False String(2:"" ("false string"), 3:"OUT_SP_00_" ("format string"), 4:"Combo Box 3") -> (0:w215:bool)  [unwired: 1 out]
            n186 = case shown="True" w215 {
              tunnel: [w220 w223] -> w216
              tunnel: "Combo Box 3" -> [w220 w222]
              frame False {
              }
              frame True {
                n187 = Number To Decimal String(number="voltage or current 2") -> (decimal integer string=w225:string)  [unwired: 1 in]
                n188 = Concatenate Strings(w222, w225, "\r\n" ("string")) -> (w223:string)
              }
            }
            "string from combo 3" <- w216
            n189 = case shown="False" "write 3" {
              tunnel: [w231 w237] -> w210
              tunnel: [w232 w236] -> w212
              tunnel: w216 -> [_ w235]
              tunnel: w205 -> [w229 _]
              frame False {
                n190 = VISA Write(VISA resource name=refnum<visa-resource-name> "COM4", write buffer="VO?\n", error in (no error)=w229) -> (VISA resource name out=w232:refnum<visa-resource-name>, error out=w231:errorcluster)  [unwired: 1 out]
              }
              frame True {
                # "Write bytes to port."
                n191 = VISA Write(VISA resource name=refnum<visa-resource-name> "COM4", write buffer=w235) -> (VISA resource name out=w236:refnum<visa-resource-name>, error out=w237:errorcluster)  [unwired: 1 in, 1 out]
              }
            }
            n192 = stacked-sequence {
              tunnel: w210 -> [w228]
              tunnel: [w228] -> w211
              tunnel: w212 -> [w227]
              tunnel: [w227] -> w213
              frame #0 {
                n193 = Wait (ms)(milliseconds to wait="delay before read (ms) 3") -> ()  [unwired: 1 out]
              }
            }
            n194 = case shown="False" "read 3" {
              tunnel: w211 -> [w240 w244]
              tunnel: [w240 w248] -> w206
              tunnel: [w239 w247] -> _
              tunnel: w213 -> [w239 w246]
              tunnel: [u32 10 ("Bytes at Port") w241] -> w203
              frame False {
              }
              frame True {
                # "Read the number of bytes specified."
                n195 = property class="Instr"(reference=w246, error in=w244) -> (reference out=w245:refnum<visa-resource-name>, error out=w243:errorcluster, "Serial Settings:Number of Bytes at Serial Port"=w241:u32)
                "bytes read 3" <- w241
                n196 = VISA Read(VISA resource name=w245, byte count=w241, error in (no error)=w243) -> (VISA resource name out=w247:refnum<visa-resource-name>, read buffer=→"inverter readout":string, error out=w248:errorcluster)  [unwired: 1 out]
              }
            }
            n197 = Equal?(x=w203, y=0.0) -> (x = y?=w202:bool)
            n198 = case shown="True" w202 {
              frame False {
              }
              frame True {
                n199 = call "inverting email"() -> ()  [unwired: 11 in, 1 out]
                n200 = local write "stop reading script"(TRUE ("stop reading script")) -> ()
                n201 = local write "read 3"(FALSE ("read 3")) -> ()
              }
            }
          }
        }
        n202 = call <vilib>:"Release Semaphore.vi"("error in (no error)"=w189, "semaphore"=w190) -> ()  [unwired: 4 in, 2 out]
        n203 = local read "Quit"() -> (w200:bool)
      }
      n204 = while {
        tunnel: w52 -> [w69]
        tunnel: [w70] -> w53
        tunnel: w43 -> [w58]
        stop <- w68 stop-if-true
        n205 = local read "COMBO COMMAND"() -> (w60:string)
        n206 = call <vilib>:"Acquire Semaphore.vi"("semaphore"=w58) -> ("error out"=w57:errorcluster, "semaphore out"=w56:T3)  [unwired: 4 in, 1 out]
        n207 = Search and Replace String(input string=w60, search string="setChiller", replace string="True" ("replace string (\"\")")) -> (result string=w65:string)  [unwired: 5 in, 3 out]
        n208 = case shown="\"False\", Default" w65 {
          tunnel: [FALSE TRUE] -> w66
          frame "False", Default {
          }
          frame "True" {
          }
        }
        n209 = local read "Quit"() -> (w67:bool)
        n210 = Or(x=w66, y=w67) -> (x .or. y?=w62:bool)
        n211 = Not(x=w62) -> (.not. x?=w61:bool)
        n212 = case shown="True" w61 {
          tunnel: [w74 w92] -> w70
          tunnel: w69 -> [w74 w91]
          tunnel: w57 -> [w73 w76]
          tunnel: [w73 w75] -> w55
          frame False {
          }
          frame True {
            # "CHILLER"
            # "Configure Serial port (baud rate,\ndata bits, parity, stop bits and flow control)."
            n213 = Match True/False String(2:"" ("false string"), 3:"OUT_SP_00_" ("format string"), 4:"Combo Box") -> (0:w84:bool)  [unwired: 1 out]
            n214 = case shown="False" w84 {
              tunnel: [w95 w98] -> w81
              tunnel: "Combo Box" -> [w95 w97]
              frame False {
              }
              frame True {
                n215 = Number To Decimal String(number="Temperature") -> (decimal integer string=w100:string)  [unwired: 1 in]
                n216 = Concatenate Strings(w97, w100, "\r\n" ("string")) -> (w98:string)
              }
            }
            "string from combo" <- w81
            n217 = case shown="False" "write" {
              tunnel: [w105 w112] -> w89
              tunnel: w91 -> [w108 w111]
              tunnel: [w106 w110] -> w87
              tunnel: w81 -> [_ w109]
              tunnel: w76 -> [w104 _]
              frame False {
                n218 = VISA Write(VISA resource name=w108, write buffer="IN_PV_00\r\n", error in (no error)=w104) -> (VISA resource name out=w106:refnum<visa-resource-name>, error out=w105:errorcluster)  [unwired: 1 out]
              }
              frame True {
                # "Write bytes to port."
                n219 = VISA Write(VISA resource name=w111, write buffer=w109) -> (VISA resource name out=w110:refnum<visa-resource-name>, error out=w112:errorcluster)  [unwired: 1 in, 1 out]
              }
            }
            n220 = stacked-sequence {
              tunnel: w89 -> [w103]
              tunnel: [w103] -> w88
              tunnel: w87 -> [w102]
              tunnel: [w102] -> w86
              frame #0 {
                n221 = Wait (ms)(milliseconds to wait="delay before read (ms)") -> ()  [unwired: 1 out]
              }
            }
            n222 = case shown="False" "read" {
              tunnel: w88 -> [w115 w120]
              tunnel: [w115 w124] -> w75
              tunnel: [w114 w123] -> w92
              tunnel: w86 -> [w114 w122]
              tunnel: [u32 10 ("return count") w116] -> w78
              frame False {
              }
              frame True {
                # "Read the number of bytes specified."
                n223 = property class="Instr"(reference=w122, error in=w120) -> (reference out=w121:refnum<visa-resource-name>, error out=w119:errorcluster, "Serial Settings:Number of Bytes at Serial Port"=w118:u32)
                "bytes read" <- w118
                n224 = VISA Read(VISA resource name=w121, byte count=w118, error in (no error)=w119) -> (VISA resource name out=w123:refnum<visa-resource-name>, read buffer=→"chiller readout (temp)":string, return count=w116:u32, error out=w124:errorcluster)
              }
            }
            n225 = Equal?(x=w78, y=0.0) -> (x = y?=w77:bool)
            n226 = case shown="True" w77 {
              frame False {
              }
              frame True {
                n227 = call "Chilling Email"() -> ()  [unwired: 11 in, 1 out]
                n228 = local write "stop reading script"(TRUE ("stop reading script")) -> ()
                n229 = local write "read"(FALSE ("read")) -> ()
              }
            }
          }
        }
        n230 = local read "Quit"() -> (w68:bool)
        n231 = Wait Until Next ms Multiple(millisecond multiple=u32 1000) -> ()  [unwired: 1 out]
        n232 = call <vilib>:"Release Semaphore.vi"("error in (no error)"=w55, "semaphore"=w56) -> ()  [unwired: 4 in, 2 out]
      }
      n233 = while {
        stop <- w622 stop-if-true
        # "dew point"
        # "N2 flow temperature"
        # "Convert text file string to array"
        # "Return the Number of lines."
        # "Extract only the size dimension we need"
        # "Get the size of the array"
        # "Read Text File, dialog box if none"
        n234 = case shown="True" "read \nrotronic log \nmanually" {
          tunnel: [w661 "File Path of rotonic datalog"] -> w620
          frame False {
            n235 = Get Date/Time In Seconds() -> (seconds since 1Jan1904=w660:timestamp)
            n236 = Format Date/Time String(time format string (%c)="%Y%m%d.xls", seconds (now)=w660) -> (date/time string=w658:string)  [unwired: 1 in]
            n237 = Concatenate Strings("C:\\Users\\CMSOTDSF.CERN\\Desktop\\rotronic_readout\\humidity_" ("time format string (%c)"), w658) -> (w662:string)
            n238 = String To Path(string=w662) -> (path=w661:path)
          }
          frame True {
          }
        }
        n239 = local read "Quit"() -> (w622:bool)
        n240 = Read from Text File(file (use dialog)=w620) -> (text=w649:string)  [unwired: 1 in, 5 out]
        n241 = Spreadsheet String To Array(delimiter (Tab)="\r", format string="%d", spreadsheet string=w649) -> (array=w647:dbl[][])  [unwired: 1 out]
        n242 = Array Size(array=w647) -> (size(s)=w648:i32[])
        n243 = Index Array(array=w648) -> (element=w651:i32)  [unwired: 1 in]
        n244 = Read from Text File(file (use dialog)=w620, count=w651) -> (text=w652:string[])  [unwired: 1 in, 4 out]
        n245 = Decrement(x=w651) -> (x-1=w650:i32)
        n246 = Array Subset(array=w652, index=w650) -> (w653:string[])  [unwired: 1 in]
        "time humidity temporature dewpoint" <- w653
        n247 = Get Date/Time In Seconds() -> (seconds since 1Jan1904=w645:timestamp)
        n248 = Array To Spreadsheet String(array=w653, 3:"%d/%m/%Y %H:%M:%S %4.12f %4.12f %4.12f" ("time format string (%c)")) -> (spreadsheet string=w624:string)  [unwired: 1 in]
        n249 = Format Date/Time String(time format string (%c)="%d/%m/%Y %H:%M:%S ", seconds (now)=w645) -> (date/time string=w646:string)  [unwired: 1 in]
        n250 = String Subset(string=w624, offset (0)=20, length (rest)=5 ("length (rest)")) -> (substring=→"humidity":string)
        n251 = Scan From String(format string=w646, input string=w624) -> (remaining string=w654:string)  [unwired: 4 in, 2 out]
        n252 = String Subset(string=w624, offset (0)=27, length (rest)=5 ("length (rest)")) -> (substring=→"temperature":string)
        n253 = String Subset(string=w624, offset (0)=34, length (rest)=6 ("length (rest)")) -> (substring=w623:string)
        "dewpoint" <- w623
        n254 = property class="Variable Object" props=["ClassId"](reference=w623) -> ()  [unwired: 1 in, 3 out]
        n255 = String Subset(string=w654, offset (0)=12, length (rest)=5 ("length (rest)")) -> (substring=w655:string)
        "dewpoint" <- w655
        n256 = Fract/Exp String To Number(string=w655) -> (number=w635:dbl)  [unwired: 3 in, 1 out]
        n257 = String Subset(string=w654, offset (0)=6, length (rest)=5 ("length (rest)")) -> (substring=w633:string)
        "n2 flow temperature" <- w633
        n258 = Fract/Exp String To Number(string=w633) -> (number=w656:dbl)  [unwired: 3 in, 1 out]
        n259 = Add(x=w635, y=5.0) -> (x+y=w634:dbl)
        n260 = Greater?(x=w656, y=w634) -> (0:→"N2 temperature > dew point + 5C":bool)
        n261 = call <vilib>:"Simple Error Handler.vi"() -> ()  [unwired: 5 in, 5 out]
      }
      n262 = while {
        stop <- w320 stop-if-true
        n263 = local read "file path (dialog if empty) 2"() -> (w321:path)
        n264 = Equal?(x=w321, y=path "") -> (x = y?=w325:bool)
        n265 = case shown="False" w325 {
          tunnel: [w327 path "C:/LabVIEW/OuterTrackerControl/example_commands.csv"] -> w326
          tunnel: w321 -> [w327 _]
          frame False {
          }
          frame True {
          }
        }
        n266 = local read "Quit"() -> (w320:bool)
        n267 = call-poly <vilib>:"Read Delimited Spreadsheet.vi"("file path (dialog if empty)"=w326, "delimiter (\\t)"="," ("delimiter (\\t)")) -> ("all rows"=w324:string[][])  [unwired: 8 in, 5 out]
        n268 = local write "all rows"(w324) -> ()
      }
      n269 = while {
        stop <- w332 stop-if-true
        w347 = u16 0 items=["Volts", "Current", "Resistance"]  # Function (0: Volts)
        w354 = u16 2 items=["Volts", "Current", "Resistance"]  # Function (0: Volts)
        w355 = u16 1 items=["Volts", "Current", "Resistance"]  # Function (0: Volts)
        # "Take the readings."
        # "Configure the output."
        # "Configure each of the three measurements. settings"
        n270 = call "Configure Measurement.vi"("Manual Range (1.0)"="Voltage Manual Range (1.0) 2", "Enable Auto Range (T:Enable)"="Enable Voltage Auto Range (T:Enable) 2", "Function (0: Volts)"=w347, "VISA resource name"=refnum<visa-resource-name> "COM1") -> ("error out"=w358:errorcluster, "VISA resource name out"=w359:refnum<visa-resource-name>)  [unwired: 6 in]
        n271 = call "Configure Measurement.vi"("Manual Range (1.0)"="Current Manual Range (1.0) 2", "error in (no error)"=w358, "Enable Auto Range (T:Enable)"="Enable Current Auto Range (T:Enable) 2", "Function (0: Volts)"=w355, "VISA resource name"=w359) -> ("error out"=w357:errorcluster, "VISA resource name out"=w356:refnum<visa-resource-name>)  [unwired: 5 in]
        n272 = call "Configure Measurement.vi"("Manual Range (1.0)"="Resistance Manual Range (1.0) 2", "error in (no error)"=w357, "Enable Auto Range (T:Enable)"="Enable Resistance Auto Range (T:Enable) 2", "Function (0: Volts)"=w354, "VISA resource name"=w356) -> ("error out"=w336:errorcluster, "VISA resource name out"=w337:refnum<visa-resource-name>)  [unwired: 5 in]
        n273 = call "Enable Output.vi"("error in (no error)"=w336, "Enable Output (T: Enable)"=TRUE, "VISA resource name"=w337) -> ("error out"=w340:errorcluster, "VISA resource name out"=w339:refnum<visa-resource-name>)  [unwired: 7 in]
        n274 = local read "COMBO COMMAND"() -> (w329:string)
        n275 = call-poly "Read.vi"("VISA resource name"=w339, "error in (no error)"=w340) -> ("Voltage"=→"Voltage 3":sgl, "Current"=w345:sgl, "Resistance"=→"Resistance 2":sgl)  [unwired: 7 in, 4 out]
        "Current 3" <- w345
        n276 = Search and Replace String(input string=w329, search string="keithleynew", replace string="1" ("replace string (\"\")")) -> (result string=w333:string)  [unwired: 5 in, 3 out]
        n277 = Multiply(x=w345, y=sgl 1000000.0) -> (x*y=→"Current Micro 2":sgl)
        n278 = case shown="\"False\", Default" w333 {
          tunnel: [FALSE TRUE] -> w331
          frame "False", Default {
            n279 = Wait (ms)(milliseconds to wait=u32 4000) -> ()  [unwired: 1 out]
          }
          frame "True" {
            n280 = Wait (ms)(milliseconds to wait=u32 4000) -> ()  [unwired: 1 out]
          }
        }
        n281 = local read "Quit"() -> (w330:bool)
        n282 = Or(x=w330, y=w331) -> (x .or. y?=w332:bool)
      }
    }
    frame #2 {
      # "Closing things down"
      n283 = VISA Close(VISA resource name=w668) -> (error out=w669:errorcluster)  [unwired: 1 in]
      "LV TTi" <- w669
      n284 = VISA Close(VISA resource name=refnum<visa-resource-name> "GPIB0::8::INSTR") -> ()  [unwired: 1 in, 1 out]
      n285 = call <vilib>:"Simple Error Handler.vi"("error in (no error)"=w669) -> ()  [unwired: 4 in, 5 out]
      n286 = VISA Close(VISA resource name=refnum<visa-resource-name> "COM4") -> (error out=w670:errorcluster)  [unwired: 1 in]
      "relay TTi" <- w670
      n287 = VISA Close(VISA resource name=w667) -> (error out=w671:errorcluster)  [unwired: 1 in]
      "Chiller" <- w671
      n288 = call <vilib>:"Simple Error Handler.vi"("error in (no error)"=w670) -> ()  [unwired: 4 in, 5 out]
      n289 = call <vilib>:"Simple Error Handler.vi"("error in (no error)"=w671) -> ()  [unwired: 4 in, 5 out]
    }
  }
  n290 = property on="dewpoint" class="Str"("Text.FontSize"=u32 30 ("Text.Font:Size")) -> ()  [unwired: 2 in, 2 out]
